vi "Set Entity Name.vi"(10 "Entity Name":string, 11 "RelationPanel in":refnum<class "RelationPanel.lvclass">) -> (3 "RelationPanel out":refnum<class "RelationPanel.lvclass">)   [LabVIEW 2020, in "Conditum-Tools.lvlib" / "RelationPanel.lvclass"]
uses:
  RelationPanel.lvclass
  RelationPanel.lvclass/RelationPanel.ctl
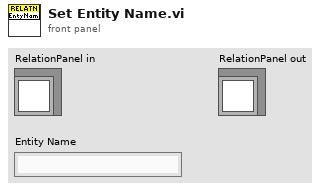
[diagram p1: front panel]
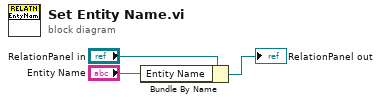
[diagram p0: block diagram]
diagram:
  n1 = Bundle By Name(cluster="RelationPanel in", "Entity Name"="Entity Name") -> (→"RelationPanel out":refnum<class "RelationPanel.lvclass">)
